vi "SAR and DSA Module Synchronization Demo.vi"() -> ()   [LabVIEW 2025]
uses:
  <vilib>/Utility/error.llb/DialogType.ctl
  <vilib>/DAQmx/write.llb/DAQmx Write (Analog Wfm 1Chan NSamp).vi
  <vilib>/DAQmx/read.llb/DAQmx Read (Analog 1D Wfm NChan NSamp).vi
  <vilib>/DAQmx/create/channels.llb/DAQmx Create Channel (AO-Voltage-Basic).vi
  <vilib>/DAQmx/configure/timing.llb/DAQmx Timing (Sample Clock).vi
  <vilib>/DAQmx/miscellaneous.llb/DAQmx Fill In Error Info.vi
  <vilib>/DAQmx/create/channels.llb/DAQmx Create Channel (AI-Voltage-Basic).vi
  <vilib>/DAQmx/configure/task.llb/DAQmx Configure Logging (TDMS).vi
  <resource>/objmgr/daqmx.rc
  <vilib>/measure/NI_MABase.lvlib
panel:
  out "AO Waveform Graph":waveform(dbl)(graph)
  out "Actual AO Sample Rate":dbl=1000.0 format="%0.2f"
  in  "Stop":bool
  out "Acquired Data Graph":waveform(dbl)[](graph)
  out "Actual AI Sample Rate":dbl
  out "error out":errorcluster
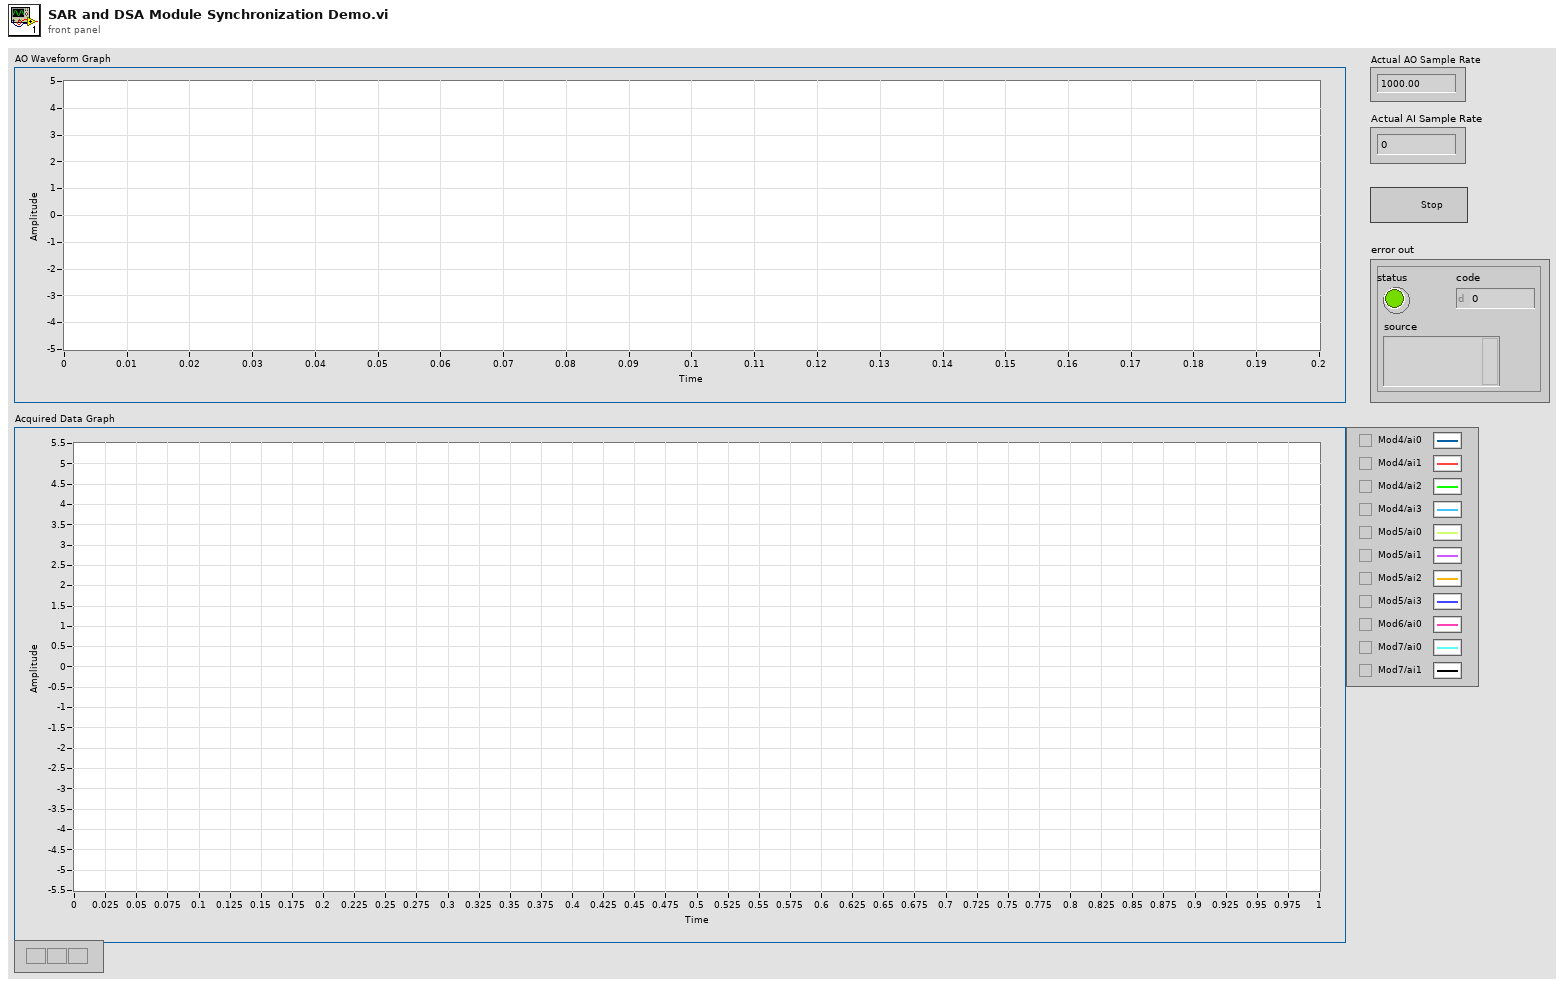
[diagram p1: front panel]
types:
  T1 = typedef "DialogType.ctl" = u16
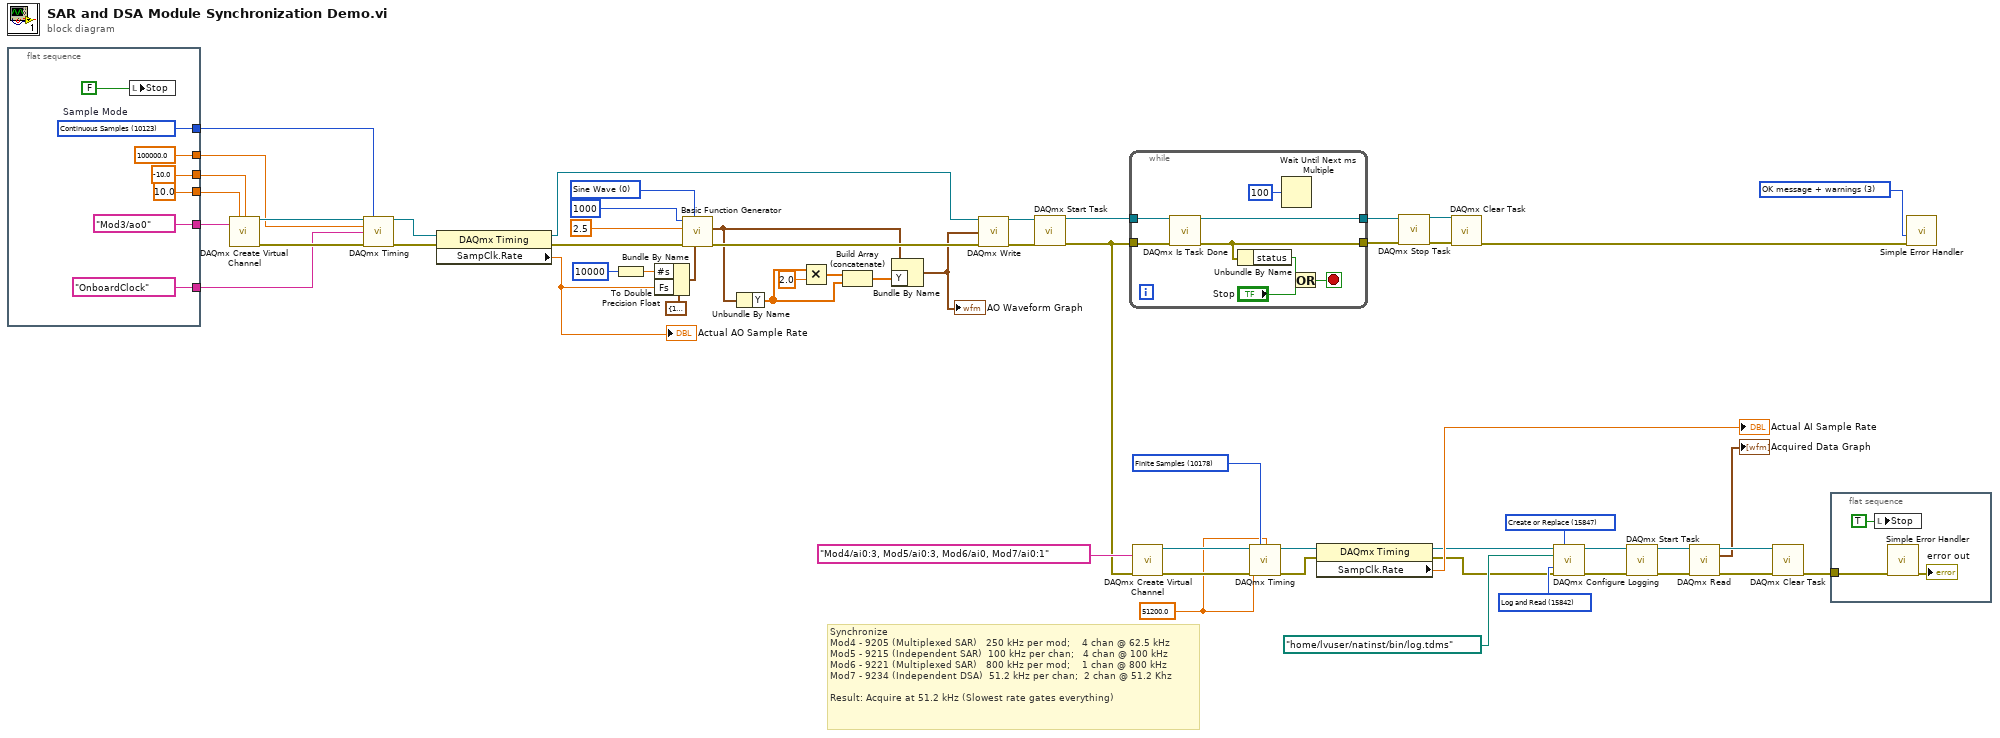
[diagram p0: block diagram]
diagram:
  w7 = 15842 items=["Off"=10231, "Log and Read"=15842] ("Logging Mode")
  w5 = 15847 items=["Open"=10437, "Open or Create"=15846, "Create or Replace"=15847, "Create"=15848] ("Operation")
  w16 = u16 0 items=["Sine Wave", "Triangle Wave", "Square Wave", "Sawtooth Wave"] ("Waveform Type")
  w29 = T1 3 items=["no dialog", "OK message", "continue or stop message", "OK message + warnings", "continue/stop + warnings"] ("type of dialog (OK msg:1)")
  w46 = 51200.0 ("rate")
  w55 = 10178 items=["Finite Samples"=10178, "Continuous Samples"=10123, "Hardware Timed Single Point"=12522] ("sample mode")
  # "Synchronize\nMod4 - 9205 (Multiplexed SAR)   250 kHz per mod;    4 chan @ 62.5 kHz\nMod5 - 9215 (Independent SAR)  100 kHz per chan;   4 chan @ 100 kHz\nMod6 - 9221 (Multiplexed SAR)   800 kHz per mod;    1 chan @ 800 kHz\nMod7 - 9234 (Independent DSA)  51.2 kHz per chan;  2 chan @ 51.2 Khz\n\nResult: Acquire at 51.2 kHz (Slowest rate gates everything)"
  n1 = flat-sequence {
    tunnel: [tag "Mod3/ao0" ("Pure Tone Channel")] -> w26
    tunnel: [-10.0 ("Min Voltage")] -> w25
    tunnel: [10.0 ("Max Voltage")] -> w24
    tunnel: [tag "OnboardClock" ("Sample Clock Source")] -> w23
    tunnel: [100000.0 ("Sample Rate")] -> w22
    tunnel: [w59] -> w21
    frame #0 {
      w59 = 10123 items=["Finite Samples"=10178, "Continuous Samples"=10123, "Hardware Timed Single Point"=12522]  # Sample Mode
      n2 = local write "Stop"(FALSE ("stop")) -> ()
    }
  }
  n3 = call-poly <vilib>:"DAQmx Create Virtual Channel.vi"("maximum value"=w24, "minimum value"=w25, "physical channels"=w26) -> ("task out"=w42:refnum<k21>, "error out"=w43:errorcluster)  [unwired: 11 in]
  n4 = call-poly <vilib>:"DAQmx Timing.vi"("task/channels in"=w42, "sample mode"=w21, "rate"=w22, "source"=w23, "error in"=w43) -> ("task out"=w20:refnum<k21>, "error out"=w44:errorcluster)  [unwired: 9 in]
  n5 = property class="DAQmx Timing"(reference=w20, error in=w44) -> (reference out=w27:refnum<k21>, error out=w28:errorcluster, "SampClk.Rate"=w38:dbl)
  "Actual AO Sample Rate" <- w38
  n6 = To Double Precision Float(number=10000 ("Number of Samples")) -> (double precision float=w35:dbl)
  n7 = Bundle By Name(cluster=cluster{"Fs":dbl, "#s":dbl} {"Fs"=1000.0, "#s"=1000.0} ("sampling info"), "#s"=w35, "Fs"=w38) -> (w15:cluster{"Fs":dbl, "#s":dbl})
  n8 = call <vilib>:"Basic Function Generator.vi"("sampling info"=w15, "signal type"=w16, "error in (no error)"=w28, "amplitude"=2.5 ("Amplitude"), "frequency"=1000 ("Frequency")) -> ("error out"=w14:errorcluster, "signal out"=w10:waveform(dbl))  [unwired: 4 in, 1 out]
  n9 = Unbundle By Name(w10) -> ("Y"=w13:dbl[])
  n10 = Multiply(x=w13, y=2.0) -> (x*y=w11:dbl[])
  n11 = Build Array (concatenate)(w11, w13) -> (w9:dbl[])
  n12 = Bundle By Name(cluster=w10, "Y"=w9) -> (w8:waveform(dbl))
  "AO Waveform Graph" <- w8
  n13 = call-poly <vilib>:"DAQmx Write.vi"("task/channels in"=w27, "data"=w8, "error in"=w14) -> ("task out"=w37:refnum<k21>, "error out"=w36:errorcluster)  [unwired: 10 in, 1 out]
  n14 = call <vilib>:"DAQmx Start Task.vi"("task/channels in"=w37, "error in"=w36) -> ("task out"=w41:refnum<k21>, "error out"=w18:errorcluster)  [unwired: 12 in]
  n15 = while {
    tunnel: w41 -> [w73]
    tunnel: w18 -> [w72]
    tunnel: [w69] -> w30
    tunnel: [w70] -> w31
    stop <- w71 stop-if-true
    n16 = call <vilib>:"DAQmx Is Task Done.vi"("task/channels in"=w73, "error in"=w72) -> ("task out"=w70:refnum<k21>, "error out"=w69:errorcluster)  [unwired: 11 in, 1 out]
    n17 = Unbundle By Name(w69) -> ("status"=w68:bool)
    n18 = Wait Until Next ms Multiple(millisecond multiple=u32 100) -> ()  [unwired: 1 out]
    n19 = Or(x=w68, y="Stop") -> (x .or. y?=w71:bool)
  }
  n20 = call-poly <vilib>:"DAQmx Create Virtual Channel.vi"("physical channels"=tag "Mod4/ai0:3, Mod5/ai0:3, Mod6/ai0, Mod7/ai0:1", "error in"=w18) -> ("task out"=w57:refnum<k21>, "error out"=w56:errorcluster)  [unwired: 12 in]
  n21 = call-poly <vilib>:"DAQmx Timing.vi"("task/channels in"=w57, "sample mode"=w55, "samples per channel"=w46, "rate"=w46, "error in"=w56) -> ("task out"=w54:refnum<k21>, "error out"=w48:errorcluster)  [unwired: 9 in]
  n22 = property class="DAQmx Timing"(reference=w54, error in=w48) -> (reference out=w4:refnum<k21>, error out=w2:errorcluster, "SampClk.Rate"=→"Actual AI Sample Rate":dbl)
  n23 = call <vilib>:"DAQmx Stop Task.vi"("task/channels in"=w31, "error in"=w30) -> ("task out"=w33:refnum<k21>, "error out"=w32:errorcluster)  [unwired: 12 in]
  n24 = call <vilib>:"DAQmx Clear Task.vi"("task in"=w33, "error in"=w32) -> ("error out"=w40:errorcluster)  [unwired: 13 in]
  n25 = call-poly <vilib>:"DAQmx Configure Logging.vi"("task/channels in"=w4, "operation"=w5, "file path"=path "/home/lvuser/natinst/bin/log.tdms" ("TDMS File Path"), "logging mode"=w7, "error in"=w2) -> ("task out"=w3:refnum<k21>, "error out"=w1:errorcluster)  [unwired: 9 in]
  n26 = call <vilib>:"DAQmx Start Task.vi"("task/channels in"=w3, "error in"=w1) -> ("task out"=w53:refnum<k21>, "error out"=w52:errorcluster)  [unwired: 12 in]
  n27 = call-poly <vilib>:"DAQmx Read.vi"("task/channels in"=w53, "error in"=w52) -> ("task out"=w51:refnum<k21>, "data"=→"Acquired Data Graph":waveform(dbl)[], "error out"=w50:errorcluster)  [unwired: 11 in]
  n28 = call <vilib>:"DAQmx Clear Task.vi"("task in"=w51, "error in"=w50) -> ("error out"=w49:errorcluster)  [unwired: 13 in]
  n29 = flat-sequence {
    tunnel: w49 -> [w76]
    frame #0 {
      n30 = local write "Stop"(TRUE ("stop")) -> ()
      n31 = call <vilib>:"Simple Error Handler.vi"("error in (no error)"=w76) -> ("error out"=→"error out":errorcluster)  [unwired: 4 in, 4 out]
    }
  }
  n32 = call <vilib>:"Simple Error Handler.vi"("type of dialog (OK msg:1)"=w29, "error in (no error)"=w40) -> ()  [unwired: 3 in, 5 out]
